vi "Vision RIO Read Time.vi"() -> (3 "Rio Talking":bool)   [LabVIEW 2020]
uses:
  <vilib>/Rock Robotics/Network Tables/NT Read Number.vi
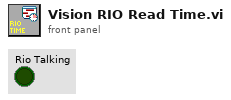
[diagram p1: front panel]
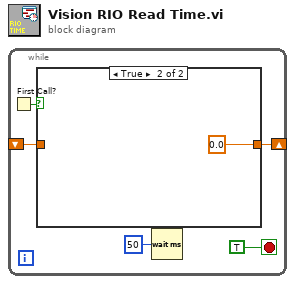
[diagram p0: block diagram]
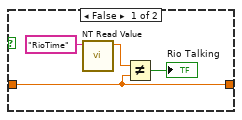
[diagram p2: hidden frame]
diagram:
  n1 = while {
    shift-right: [w4] -> _
    shift-left: _ -> [w3]
    stop <- TRUE stop-if-true
    n2 = First Call?() -> (First Call?: T/F=w5:bool)
    n3 = case shown="True" w5 {
      tunnel: [w7 0.0] -> w4
      tunnel: w3 -> [w7 _]
      frame False {
        n4 = call-poly <vilib>:"NT Read Value.vi"("Name"="RioTime") -> ("Numeric"=w8:dbl)  [unwired: 9 in, 1 out]
        n5 = Not Equal?(x=w8, y=w7) -> (x != y?=→"Rio Talking":bool)
      }
      frame True {
      }
    }
    n6 = Wait (ms)(milliseconds to wait=u32 50) -> ()  [unwired: 1 out]
  }
